vi "Get Now Playing Info.vi"() -> ()   [LabVIEW 2013]
uses:
  Private/Type Defs/JSON/List.Fields.All.ctl
  LVH-XBMC.lvlib
  Public/Player/Player.lvlib
panel:
  out "Value 2":string[](array[string])
  out "Value":string
  in  "Properties":T1[](array[typedef])
  out "Error Out":errorcluster
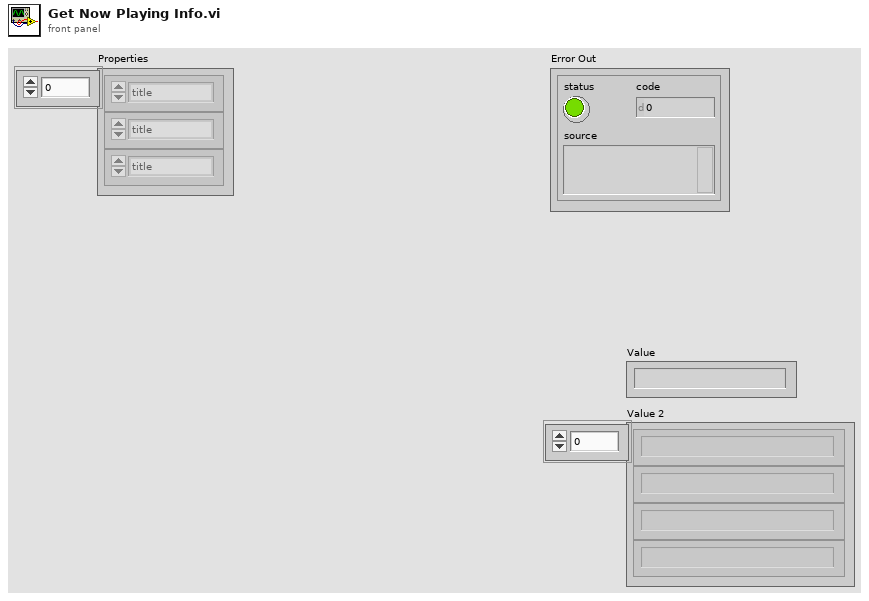
[diagram p1: front panel]
types:
  T1 = typedef "LVH-XBMC.lvlib/List.Fields.All.ctl" = enum16{"title", "artist", "albumartist", "genre", "year", "rating", "album", "track", "duration", "comment", "lyrics", "musicbrainztrackid", "musicbrainzartistid", "musicbrainzalbumid", "musicbrainzalbumartistid", "playcount", "fanart", "director", "trailer", "tagline", "plot", "plotoutline", "originaltitle", "lastplayed", "writer", "studio", "mpaa", "cast", "country", "imdbnumber", "premiered", "productioncode", "runtime", "set", "showlink", "streamdetails", "top250", "votes", "firstaired", "season", "episode", "showtitle", "thumbnail", "file", "resume", "artistid", "albumid", "tvshowid", "setid", "watchedepisodes", "disc", "tag", "art", "genreid", "displayartist", "albumartistid", "description", "theme", "mood", "style", "albumlabel", "sorttitle", "episodeguide", "uniqueid", "dateadded", "channel", "channeltype", "hidden", "locked", "channelnumber", "starttime", "endtime"}
  T2 = typedef "LVH-XBMC.lvlib/XBMC Ref.ctl" = cluster{"HTTP Handle":T3, "Hostname / IP":string, "jsonrpc":string}
  T3 = typedef "LabVIEWHTTPClient.lvlib/ClientHandle.ctl" = refnum<k1>
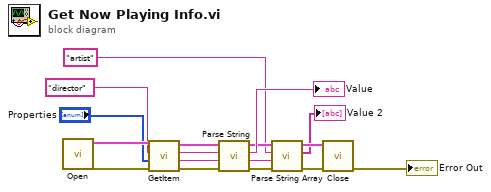
[diagram p0: block diagram]
diagram:
  n1 = call "Open.vi"() -> ("Error Out"=w15:errorcluster, "XBMC Ref"=w16:T2)  [unwired: 10 in]
  n2 = call "GetItem.vi"("Error In"=w15, "Properties"="Properties", "XBMC Ref"=w16) -> ("Error Out"=w12:errorcluster, "Response"=w10:string, "XBMC Ref"=w11:T2)  [unwired: 6 in]
  n3 = call "Parse String.vi"("Error In"=w12, "JSON Response"=w10, "Key"="director", "XBMC Ref"=w11) -> ("Error Out"=w6:errorcluster, "Dup JSON Response"=w7:string, "Value"=→"Value":string, "XBMC Ref"=w3:T2)  [unwired: 4 in]
  n4 = call "Parse String Array.vi"("Error In"=w6, "JSON Response"=w7, "Key"="artist", "XBMC Ref"=w3) -> ("Error Out"=w5:errorcluster, "Value"=→"Value 2":string[], "XBMC Ref"=w4:T2)  [unwired: 4 in, 1 out]
  n5 = call "Close.vi"("Error In"=w5, "XBMC Ref"=w4) -> ("Error Out"=→"Error Out":errorcluster)  [unwired: 9 in]
